vi "Bundle.vi"(8 "error in (no error)":errorcluster, 9 "Resistance at 0°C(100Ohm)":dbl=100.0, 10 "RTD Type":T1=enum."Pt3851" caption="RTD Type(Pt3851)", 11 "DMM Config RTD Type Msg in":refnum<class "DMM Config RTD Type Msg.lvclass">) -> (0 "error out":errorcluster, 3 "DMM Config RTD Type Msg out":refnum<class "DMM Config RTD Type Msg.lvclass">)   [LabVIEW 2020, in "DMM Msg.lvlib" / "DMM Config RTD Type Msg.lvclass"]
doc: "Populate the message class."
uses:
  DMM Config RTD Type Msg.lvclass
  PPL/HDH.Driver.DMM.lvlibp/Controls/Ctl_RTDType.ctl
  DMM Config RTD Type Msg.lvclass/DMM Config RTD Type Msg.ctl
  PPL/HDH.Driver.DMM.lvlibp
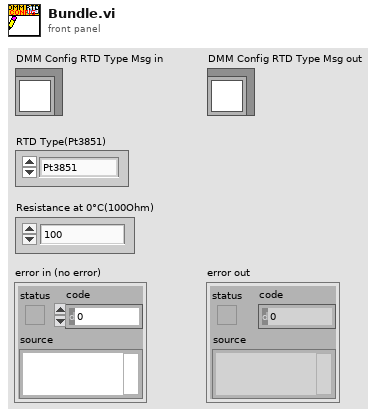
[diagram p1: front panel]
types:
  T1 = typedef "HDH.Driver.DMM.lvlibp/Ctl_RTDType.ctl" = enum16{"Custom", "Pt3750", "Pt3851", "Pt3911", "Pt3916", "Pt3920", "Pt3928"}
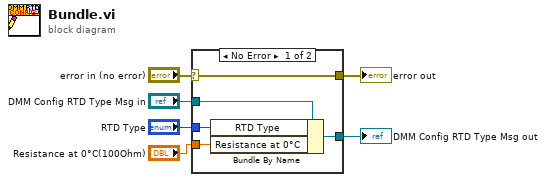
[diagram p0: block diagram]
diagram:
  n1 = case shown="No Error" "error in (no error)" {
    selector: "error in (no error)" -> [w11 w12]
    tunnel: [w11 w12] -> w5
    tunnel: [w9 w13] -> w3
    tunnel: "DMM Config RTD Type Msg in" -> [w10 w13]
    tunnel: "RTD Type" -> [w8 _]
    tunnel: "Resistance at 0°C(100Ohm)" -> [w7 _]
    frame No Error {
      n2 = Bundle By Name(cluster=w10, "RTD Type"=w8, "Resistance at 0°C"=w7) -> (w9:refnum<class "DMM Config RTD Type Msg.lvclass">)
    }
    frame Error {
    }
  }
  "error out" <- w5
  "DMM Config RTD Type Msg out" <- w3
